vi "Test Result Status Convert.vi"(1 "Result":T1) -> (0 "Result String":string)   [LabVIEW 2015, in "JsonReportPlugin.lvclass"]
uses:
  JsonReportPlugin.lvclass
  Core/Execution/EXECUTION_RESULT_TYPEDEF.ctl
  Core/Execution.lvclass
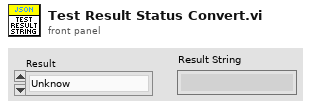
[diagram p1: front panel]
types:
  T1 = typedef "Execution.lvclass/EXECUTION_RESULT_TYPEDEF.ctl" = enum16{"Unknow", "Terminated", "Passed", "Failed", "Error"}
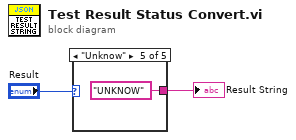
[diagram p0: block diagram]
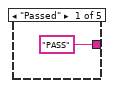
[diagram p2: hidden frame]
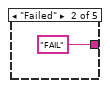
[diagram p3: hidden frame]
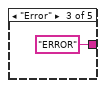
[diagram p4: hidden frame]
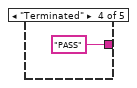
[diagram p5: hidden frame]
diagram:
  n1 = case shown="\"Unknow\"" "Result" {
    tunnel: ["PASS" "FAIL" "ERROR" "PASS" "UNKNOW"] -> w2
    frame "Passed" {
    }
    frame "Failed" {
    }
    frame "Error" {
    }
    frame "Terminated" {
    }
    frame "Unknow" {
    }
  }
  "Result String" <- w2
